vi "LM3Sxxxx_Sequence_Config.vi"(8 "error in (no error)":errorcluster, 10 "Config Data":string[](array[string]), 11 "Interrupt Name":string) -> (0 "error out":errorcluster, 3 "Interrupt Configuration":string[](array[string]))   [LabVIEW 2011]
panel:
  in  "Samples":u32(ring)=4 items=["1"=1, "2"=2, "3"=3, "4"=4]
  in  "Sample frequency":u32(ring)=512 items=["500 kHz"=512, "250 kHz"=256, "125 kHz"=0]
  in  "Sampled pin":u32(ring) items=["ADC0", "ADC1", "ADC2", "ADC3", "ADC0 and ADC1 differential", "ADC2 and ADC3 differential"]
  in  "help":bool
  in  "Priority":u32(ring)=1 items=["0", "1", "2", "3"]
  in  "cancel":bool
  in  "ok":bool
  in  "Sequence trigger":u32(ring) items=["External pin"=4, "Processor"=0, "Always"=15, "PWM 0"=6, "PWM 1"=7, "PWM 2"=8, "Timer"=5, "Comparator"=1]
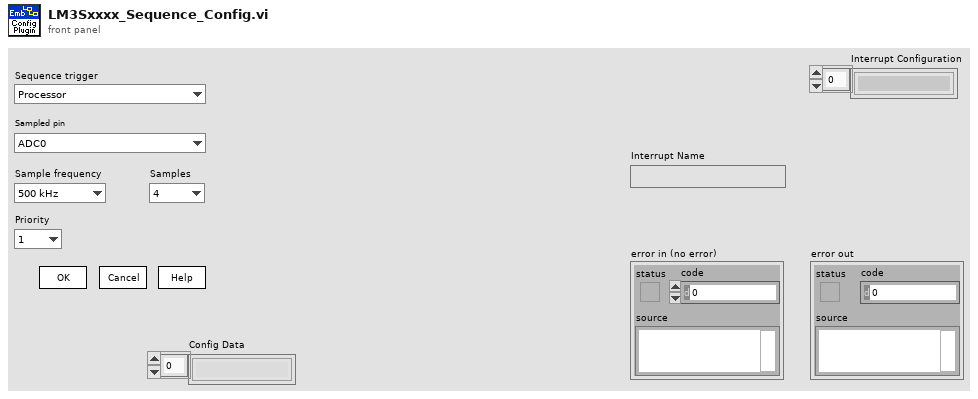
[diagram p1: front panel]
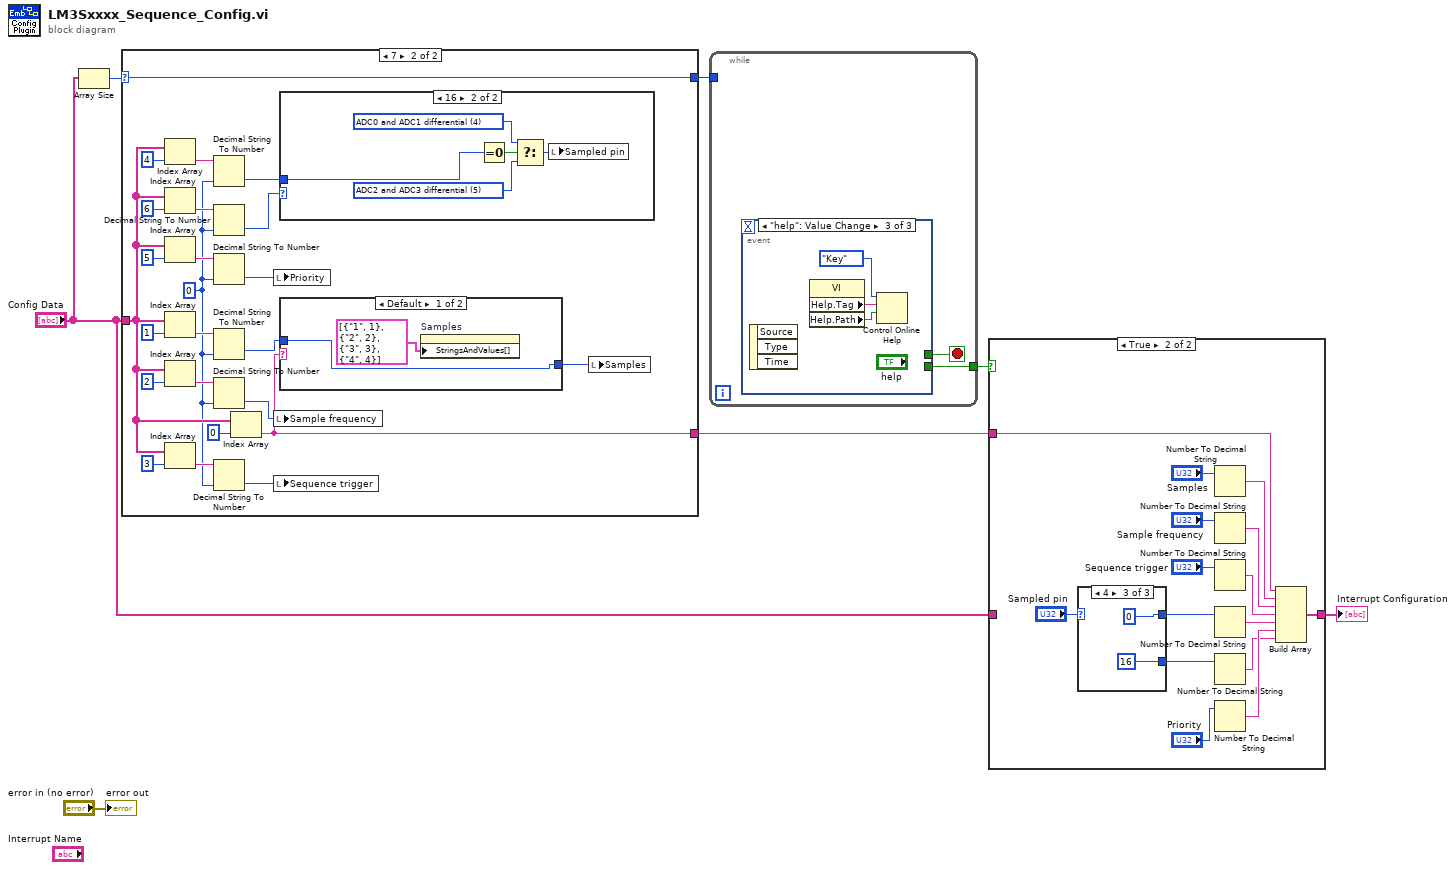
[diagram p0: block diagram]
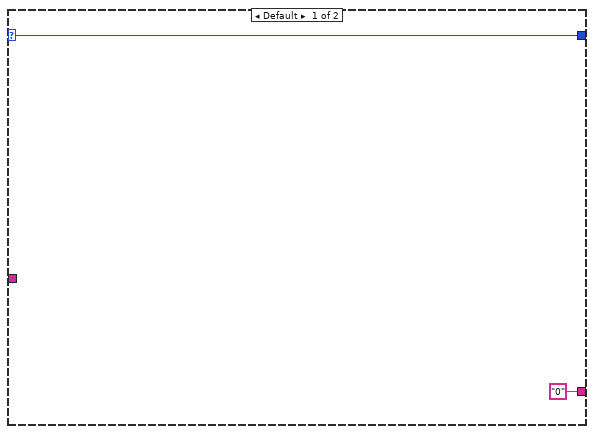
[diagram p2: hidden frame]
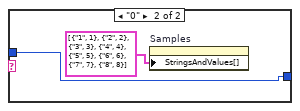
[diagram p3: hidden frame]
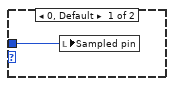
[diagram p4: hidden frame]
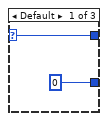
[diagram p6: hidden frame]
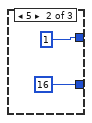
[diagram p7: hidden frame]
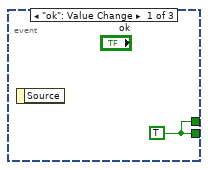
[diagram p8: hidden frame]
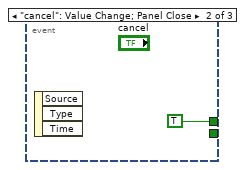
[diagram p9: hidden frame]
diagram:
  n1 = Array Size(array="Config Data") -> (size(s)=w5:i32)
  n2 = case shown="7" w5 {
    selector: w5 -> [w9 w33]
    tunnel: [w9 w33] -> w4
    tunnel: "Config Data" -> [_ w19]
    tunnel: ["0" ("String") w12] -> w2
    frame Default {
    }
    frame 7 {
      w16 = u32 0
      n3 = Index Array(array=w19, index=4) -> (element=w22:string)
      n4 = Index Array(array=w19, index=6) -> (element=w24:string)
      n5 = Index Array(array=w19, index=5) -> (element=w20:string)
      n6 = Index Array(array=w19, index=1) -> (element=w26:string)
      n7 = Index Array(array=w19, index=2) -> (element=w25:string)
      n8 = Index Array(array=w19, index=3) -> (element=w17:string)
      n9 = Decimal String To Number(string=w22, default (0L)=w16) -> (number=w21:u32)  [unwired: 1 in, 1 out]
      n10 = Decimal String To Number(string=w24, default (0L)=w16) -> (number=w23:u32)  [unwired: 1 in, 1 out]
      n11 = Decimal String To Number(string=w20, default (0L)=w16) -> (number=w13:u32)  [unwired: 1 in, 1 out]
      n12 = Decimal String To Number(string=w26, default (0L)=w16) -> (number=w11:u32)  [unwired: 2 out]
      n13 = Decimal String To Number(string=w25, default (0L)=w16) -> (number=w15:u32)  [unwired: 2 out]
      n14 = Decimal String To Number(string=w17, default (0L)=w16) -> (number=w14:u32)  [unwired: 2 out]
      n15 = Index Array(array=w19, index=0) -> (element=w12:string)
      n16 = local write "Priority"(w13) -> ()
      n17 = local write "Sample frequency"(w15) -> ()
      n18 = local write "Sequence trigger"(w14) -> ()
      n19 = case shown="16" w23 {
        tunnel: w21 -> [w38 w39]
        frame 0, Default {
          n20 = local write "Sampled pin"(w38) -> ()
        }
        frame 16 {
          w40 = u32 5 items=["ADC0", "ADC1", "ADC2", "ADC3", "ADC0 and ADC1 differential", "ADC2 and ADC3 differential"] ("Sampled pin")
          w41 = u32 4 items=["ADC0", "ADC1", "ADC2", "ADC3", "ADC0 and ADC1 differential", "ADC2 and ADC3 differential"] ("Sampled pin")
          n21 = Equal To 0?(x=w39) -> (x = 0?=w42:bool)
          n22 = Select(t=w41, s=w42, f=w40) -> (s? t:f=w43:u32)
          n23 = local write "Sampled pin"(w43) -> ()
        }
      }
      n24 = case shown="Default" w12 {
        tunnel: w11 -> [w34 w36]
        tunnel: [w34 w36] -> w10
        frame Default {
          n25 = property on="Samples" class="Ring (strict)"("StringsAndValues[]"=cluster{"String":string, "Value":u32}[] [{"String"="1", "Value"=1}, {"String"="2", "Value"=2}, {"String"="3", "Value"=3}, {"String"="4", "Value"=4}] ("Strings And Values []")) -> ()  [unwired: 2 in, 2 out]
        }
        frame "0" {
          n26 = property on="Samples" class="Ring (strict)"("StringsAndValues[]"=cluster{"String":string, "Value":u32}[] [{"String"="1", "Value"=1}, {"String"="2", "Value"=2}, {"String"="3", "Value"=3}, {"String"="4", "Value"=4}, {"String"="5", "Value"=5}, {"String"="6", "Value"=6}, {"String"="7", "Value"=7}, {"String"="8", "Value"=8}] ("Strings And Values []")) -> ()  [unwired: 2 in, 2 out]
        }
      }
      n27 = local write "Samples"(w10) -> ()
    }
  }
  n28 = while {
    tunnel: [w44] -> w1
    tunnel: w4 -> [_]
    stop <- w45 stop-if-true
    n29 = event shown="[2] \"help\": Value Change" {
      selector: _ -> [_ _ _]
      dyn-events: _ -> [_ _ _]
      timeout: _ -> [_ _ _]
      tunnel: [w46 TRUE _] -> w45
      tunnel: [w46 _ _] -> w44
      event "ok": Value Change {
        w46 = TRUE
        n30 = event-data() -> ()  [unwired: 2 out]
      }
      event "cancel": Value Change; Panel Close {
        n31 = event-data() -> ()  [unwired: 4 out]
      }
      event "help": Value Change {
        n32 = event-data() -> ()  [unwired: 4 out]
        n33 = property class="VI"() -> ("Help.Tag"=w48:string, "Help.Path"=w49:path)  [unwired: 2 in, 2 out]
        n34 = Control Online Help(2:w49, 3:w48, 4:enum16{"Contents", "Key", "Close"}."Key" ("Operation")) -> ()  [unwired: 1 in, 1 out]
      }
    }
  }
  n35 = case shown="True" w1 {
    tunnel: [w51 w65] -> w6
    tunnel: "Config Data" -> [w51 _]
    tunnel: w2 -> [_ w66]
    frame False {
    }
    frame True {
      n36 = case shown="4" "Sampled pin" {
        selector: "Sampled pin" -> [w68 _ _]
        tunnel: [w68 u32 1 ("Sampled pin") u32 0 ("Sampled pin")] -> w55
        tunnel: [u32 0 u32 16 u32 16] -> w52
        frame Default {
        }
        frame 5 {
        }
        frame 4 {
        }
      }
      n37 = Number To Decimal String(number="Samples") -> (decimal integer string=w64:string)  [unwired: 1 in]
      n38 = Number To Decimal String(number="Sample frequency") -> (decimal integer string=w62:string)  [unwired: 1 in]
      n39 = Number To Decimal String(number="Sequence trigger") -> (decimal integer string=w60:string)  [unwired: 1 in]
      n40 = Number To Decimal String(number=w55) -> (decimal integer string=w54:string)  [unwired: 1 in]
      n41 = Number To Decimal String(number=w52) -> (decimal integer string=w53:string)  [unwired: 1 in]
      n42 = Number To Decimal String(number="Priority") -> (decimal integer string=w57:string)  [unwired: 1 in]
      n43 = Build Array(w66, w64, w62, w60, w54, w57, w53) -> (w65:string[])
    }
  }
  "Interrupt Configuration" <- w6
  "error out" <- "error in (no error)"
